vi "Untitled 12.vi"(8 "error in (no error)":errorcluster, 11 "Visualization in":refnum<class "Visualization.lvclass">) -> (0 "error out":errorcluster, 3 "Visualization out":refnum<class "Visualization.lvclass">)   [LabVIEW 2019, in "Visualization.lvclass"]
uses:
  Visualization.lvclass
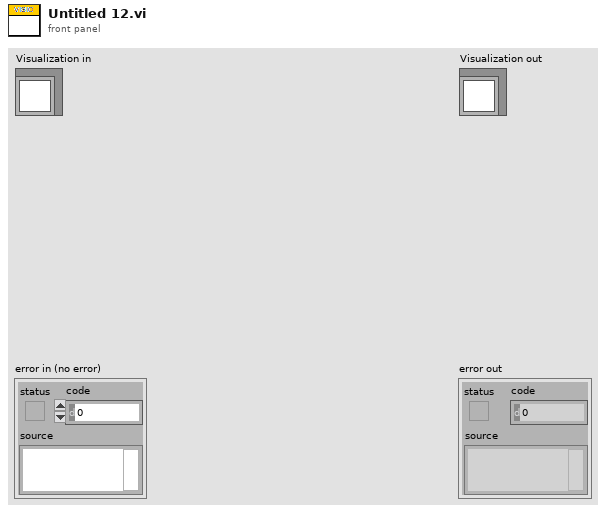
[diagram p1: front panel]
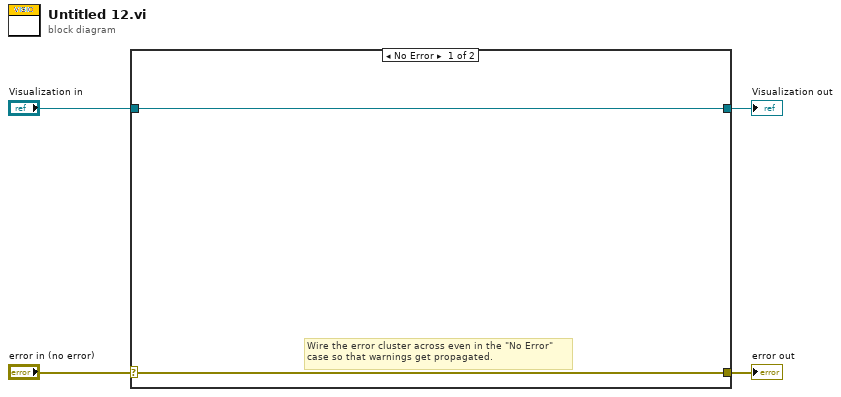
[diagram p0: block diagram]
diagram:
  n1 = case shown="No Error" "error in (no error)" {
    selector: "error in (no error)" -> [w5 w8]
    tunnel: [w5 w8] -> w3
    tunnel: [w6 w7] -> w1
    tunnel: "Visualization in" -> [w6 w7]
    frame No Error {
      # "Wire the error cluster across even in the \"No Error\"\ncase so that warnings get propagated."
    }
    frame Error {
    }
  }
  "error out" <- w3
  "Visualization out" <- w1
